vi "Queue Add.vi"(8 "错误输入（无错误）":errorcluster, 9 "消息数据":variant, 10 "消息":string, 11 "队列输入":refnum<queue>) -> (0 "错误输出":errorcluster, 3 "队列输出":refnum<queue>)   [LabVIEW 2023]
uses:
  Ctl/QMH Fundamentals - Message Cluster.ctl
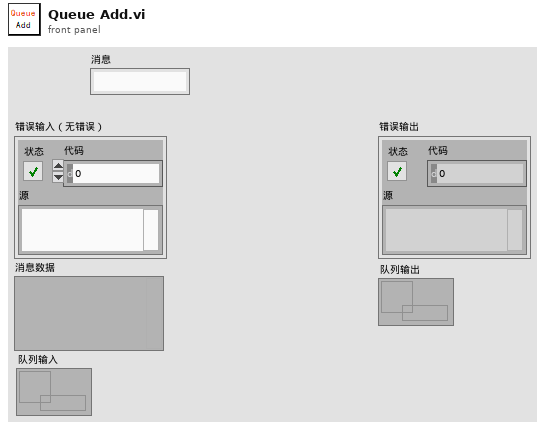
[diagram p1: front panel]
types:
  T1 = typedef "QMH Fundamentals - Message Cluster.ctl" = cluster{"消息":string, "消息数据":variant}
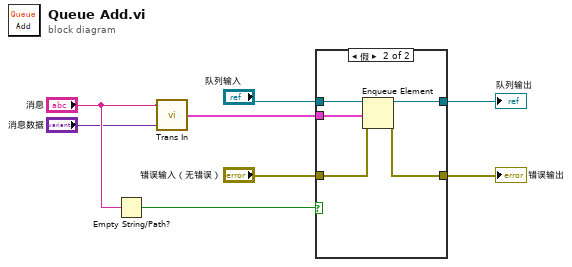
[diagram p0: block diagram]
diagram:
  n1 = Empty String/Path?(string/path="消息") -> (empty?=w6:bool)
  n2 = call "Trans In.vi"("消息数据"="消息数据", "消息"="消息") -> ("输出簇"=w3:T1)  [unwired: 1 in]
  n3 = case shown="假" w6 {
    tunnel: "队列输入" -> [w10 w15]
    tunnel: [w10 w14] -> w4
    tunnel: "错误输入（无错误）" -> [w9 w13]
    tunnel: [w9 w12] -> w7
    tunnel: w3 -> [_ w11]
    frame True {
    }
    frame False {
      n4 = Enqueue Element(queue=w15, element=w11, error in (no error)=w13) -> (queue out=w14:refnum<queue>, error out=w12:errorcluster)  [unwired: 1 in, 1 out]
    }
  }
  "错误输出" <- w7
  "队列输出" <- w4
